vi "Init.vi"(8 "error in (no error)":errorcluster, 11 "abs_EventLog in":refnum<class "abs_EventLog.lvclass">) -> (0 "error out":errorcluster, 3 "abs_EventLog out":refnum<class "abs_EventLog.lvclass">)   [LabVIEW 2021, in "abs_EventLog.lvclass"]
uses:
  abs_EventLog.lvclass
  abs_EventLog.lvclass/abs_EventLog.ctl
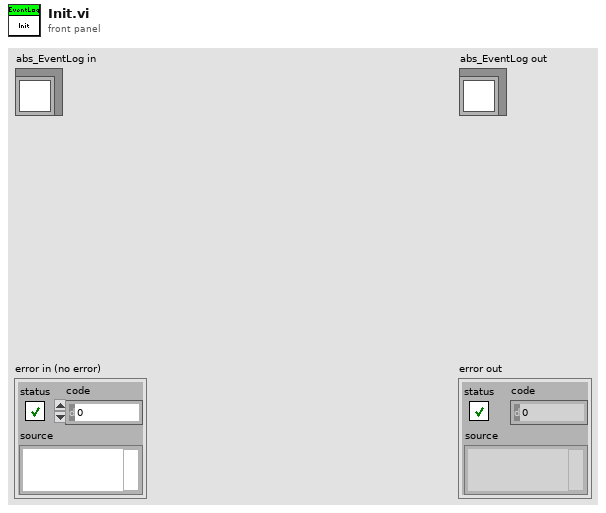
[diagram p1: front panel]
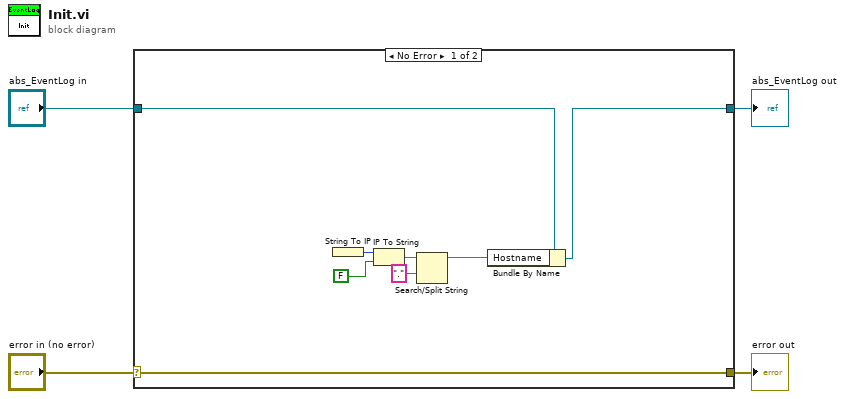
[diagram p0: block diagram]
diagram:
  n1 = case shown="No Error" "error in (no error)" {
    selector: "error in (no error)" -> [w12 w14]
    tunnel: [w12 w14] -> w3
    tunnel: [w5 w13] -> w1
    tunnel: "abs_EventLog in" -> [w7 w13]
    frame No Error {
      n2 = String To IP() -> (0:w9:u32)  [unwired: 1 in]
      n3 = IP To String(1:FALSE ("dot notation? (F)"), 2:w9) -> (0:w10:string)
      n4 = Search/Split String(string=w10, search string/char (-)=".") -> (substring before match=w6:string)  [unwired: 1 in, 2 out]
      n5 = Bundle By Name(cluster=w7, "Hostname"=w6) -> (w5:refnum<class "abs_EventLog.lvclass">)
    }
    frame Error {
    }
  }
  "error out" <- w3
  "abs_EventLog out" <- w1
